vi "toml_load.vi"(8 "error in (no error)":errorcluster, 11 "toml":string) -> (0 "error out":errorcluster, 3 "sections":T1[](array[typedef]))   [LabVIEW 2017]
uses:
  toml_fg_section.ctl
  toml_fg_row.ctl
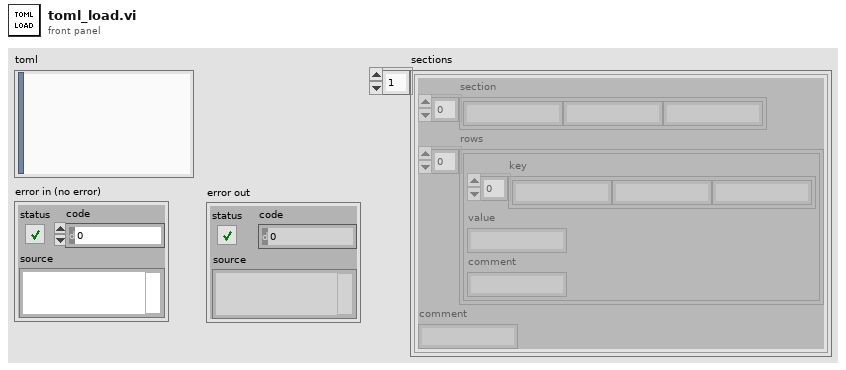
[diagram p1: front panel]
types:
  T1 = typedef "toml_fg_section.ctl" = cluster{"section":string[], "rows":T2[], "comment":string}
  T2 = typedef "toml_fg_row.ctl" = cluster{"key":string[], "value":string, "comment":string}
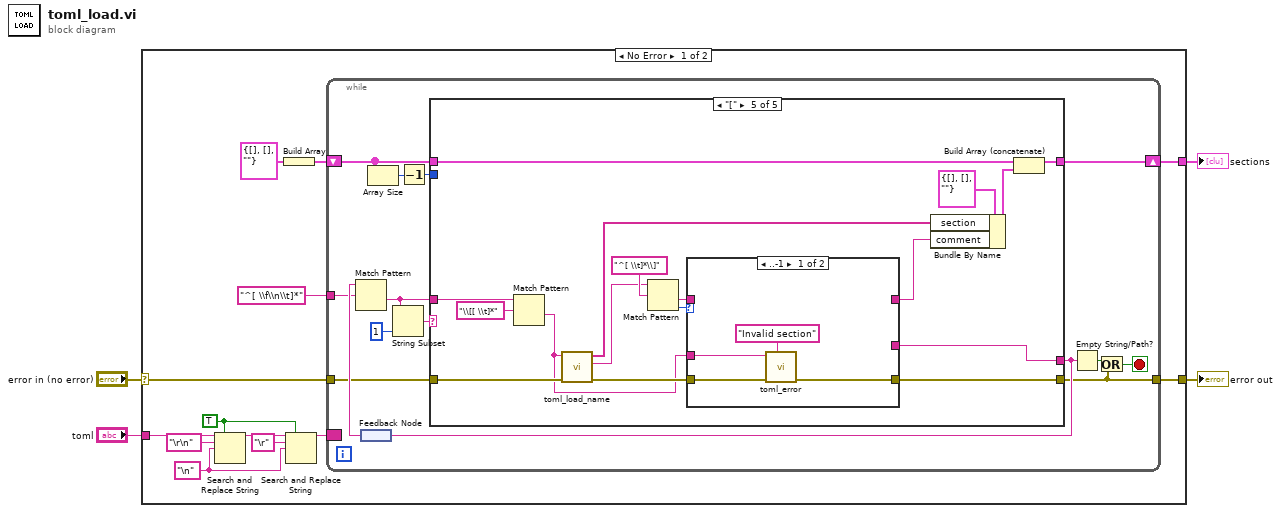
[diagram p0: block diagram]
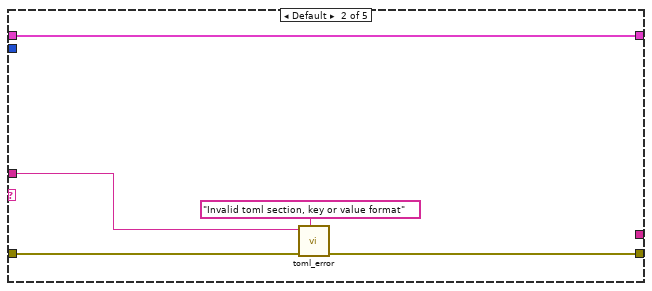
[diagram p3: hidden frame]
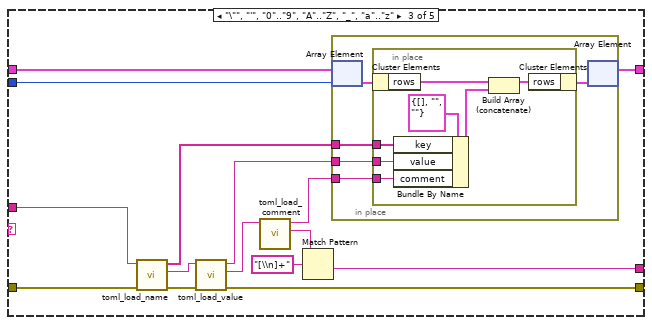
[diagram p4: hidden frame]
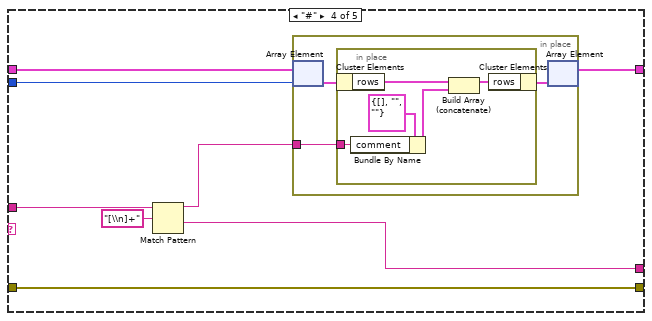
[diagram p5: hidden frame]
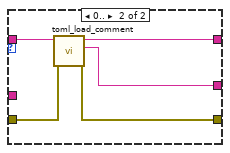
[diagram p6: hidden frame]
diagram:
  n1 = case shown="No Error" "error in (no error)" {
    selector: "error in (no error)" -> [w12 w108]
    tunnel: [w16 _] -> w4
    tunnel: "toml" -> [w14 _]
    tunnel: [w10 w108] -> w1
    frame No Error {
      w9 = "\n" ("search string")
      w8 = TRUE ("replace all? (F)")
      n2 = Search and Replace String(replace all?=w8, input string=w14, search string="\r\n", replace string=w9) -> (result string=w6:string)  [unwired: 4 in, 3 out]
      n3 = Build Array(T1 {"section"=[], "rows"=[], "comment"=""} ("section")) -> (w15:T1[])
      n4 = Search and Replace String(replace all?=w8, input string=w6, search string="\r", replace string=w9) -> (result string=w13:string)  [unwired: 4 in, 3 out]
      n5 = while {
        shift-right: [w23] -> w16
        shift-left: w15 -> [w26]
        border: w13 -> [_]
        tunnel: w12 -> [w27]
        tunnel: "^[ \\f\\n\\t]*" ("regular expression") -> [w24]
        tunnel: [w20] -> w10
        stop <- w19 stop-if-true
        n6 = feedback #1() -> (w31:string)
        n7 = Match Pattern(string=w31, regular expression=w24) -> (after substring=w28:string)  [unwired: 1 in, 3 out]
        n8 = Array Size(array=w26) -> (size(s)=w25:i32)
        n9 = String Subset(string=w28, length (rest)=1 ("length (rest)")) -> (substring=w29:string)  [unwired: 1 in]
        n10 = Decrement(x=w25) -> (x-1=w18:i32)
        n11 = case shown="\"[\"" w29 {
          tunnel: w28 -> [_ w35 w52 w73 w84]
          tunnel: w27 -> [w32 w37 w53 w66 w98]
          tunnel: w26 -> [w33 w38 w51 w70 w97]
          tunnel: w18 -> [_ _ w45 w69 _]
          tunnel: [_ _ w39 w71 w86] -> w22
          tunnel: [w33 w38 w50 w68 w96] -> w23
          tunnel: [w32 w36 w47 w66 w90] -> w20
          frame "" {
          }
          frame Default {
            n12 = call "toml_error.vi"("message"="Invalid toml section, key or value format", "error in (no error)"=w37, "toml"=w35) -> ("error out"=w36:errorcluster)  [unwired: 8 in]
          }
          frame "\"", "'", "0".."9", "A".."Z", "_", "a".."z" {
            n13 = call "toml_load_name.vi"("error in (no error)"=w53, "toml"=w52) -> ("error out"=w48:errorcluster, "remaining string"=w46:string, "name"=w49:string[])  [unwired: 7 in]
            n14 = call "toml_load_value.vi"("error in (no error)"=w48, "toml"=w46) -> ("error out"=w47:errorcluster, "remaining string"=w42:string, "value"=w40:string)  [unwired: 7 in]
            n15 = call "toml_load_comment.vi"("toml"=w42) -> ("remaining string"=w43:string, "inline comment"=w41:string)  [unwired: 8 in, 1 out]
            n16 = Match Pattern(string=w43, regular expression="[\\n]+") -> (after substring=w39:string)  [unwired: 1 in, 3 out]
            n17 = in-place {
              in-place-border: w41 -> [w57]
              in-place-border: w49 -> [w55]
              in-place-border: w40 -> [w54]
              n18 = in-place-array #2(w51, w45) -> (w58:T1)
              n19 = in-place {
                in-place-border: w57 -> [w62]
                in-place-border: w55 -> [w60]
                in-place-border: w54 -> [w59]
                n20 = in-place-cluster #3(w58) -> ("rows"=w65:T2[])
                n21 = Bundle By Name(cluster=T2 {"key"=[], "value"="", "comment"=""} ("row"), "key"=w60, "value"=w59, "comment"=w62) -> (w61:T2)
                n22 = Build Array (concatenate)(w65, w61) -> (w64:T2[])
                n23 = in-place-cluster #3("rows"=w64) -> (w56:T1)
              }
              n24 = in-place-array #2(w56) -> (w50:T1[])  [unwired: 1 out]
            }
          }
          frame "#" {
            n25 = Match Pattern(string=w73, regular expression="[\\n]+") -> (before substring=w67:string, after substring=w71:string)  [unwired: 1 in, 2 out]
            n26 = in-place {
              in-place-border: w67 -> [w75]
              n27 = in-place-array #4(w70, w69) -> (w76:T1)
              n28 = in-place {
                in-place-border: w75 -> [w78]
                n29 = in-place-cluster #5(w76) -> ("rows"=w81:T2[])
                n30 = Bundle By Name(cluster=T2 {"key"=[], "value"="", "comment"=""} ("row"), "comment"=w78) -> (w77:T2)
                n31 = Build Array (concatenate)(w81, w77) -> (w80:T2[])
                n32 = in-place-cluster #5("rows"=w80) -> (w74:T1)
              }
              n33 = in-place-array #4(w74) -> (w68:T1[])  [unwired: 1 out]
            }
          }
          frame "[" {
            n34 = Match Pattern(string=w84, regular expression="\\[[ \\t]*") -> (after substring=w83:string)  [unwired: 1 in, 3 out]
            n35 = call "toml_load_name.vi"("error in (no error)"=w98, "toml"=w83) -> ("error out"=w89:errorcluster, "remaining string"=w87:string, "name"=w85:string[])  [unwired: 7 in]
            n36 = Match Pattern(string=w87, regular expression="^[ \\t]*\\]") -> (after substring=w92:string, offset past match=w88:i32)  [unwired: 1 in, 2 out]
            n37 = case shown="..-1" w88 {
              tunnel: w92 -> [_ w106]
              tunnel: [_ w107] -> w91
              tunnel: [_ w103] -> w86
              tunnel: [w101 w104] -> w90
              tunnel: w89 -> [w102 w105]
              tunnel: w83 -> [w99 _]
              frame ..-1 {
                n38 = call "toml_error.vi"("message"="Invalid section", "error in (no error)"=w102, "toml"=w99) -> ("error out"=w101:errorcluster)  [unwired: 8 in]
              }
              frame 0.. {
                n39 = call "toml_load_comment.vi"("error in (no error)"=w105, "toml"=w106) -> ("error out"=w104:errorcluster, "remaining string"=w103:string, "inline comment"=w107:string)  [unwired: 7 in]
              }
            }
            n40 = Bundle By Name(cluster=T1 {"section"=[], "rows"=[], "comment"=""} ("section"), "section"=w85, "comment"=w91) -> (w94:T1)
            n41 = Build Array (concatenate)(w97, w94) -> (w96:T1[])
          }
        }
        n42 = feedback-in #1(w22) -> ()
        n43 = Empty String/Path?(string/path=w22) -> (empty?=w21:bool)
        n44 = Or(x=w21, y=w20) -> (x .or. y?=w19:bool)
      }
    }
    frame Error {
    }
  }
  "sections" <- w4
  "error out" <- w1
